vi "Turn To Angle.vi"(9 "Speed/Direction":dbl, 10 "Angle":dbl, 11 "drive.lvclass":refnum<class "drive.lvclass">) -> (3 "drive.lvclass":refnum<class "drive.lvclass">)   [LabVIEW 2015, in "drive.lvclass"]
uses:
  drive.lvclass
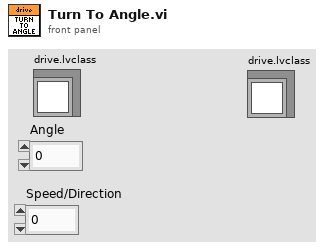
[diagram p1: front panel]
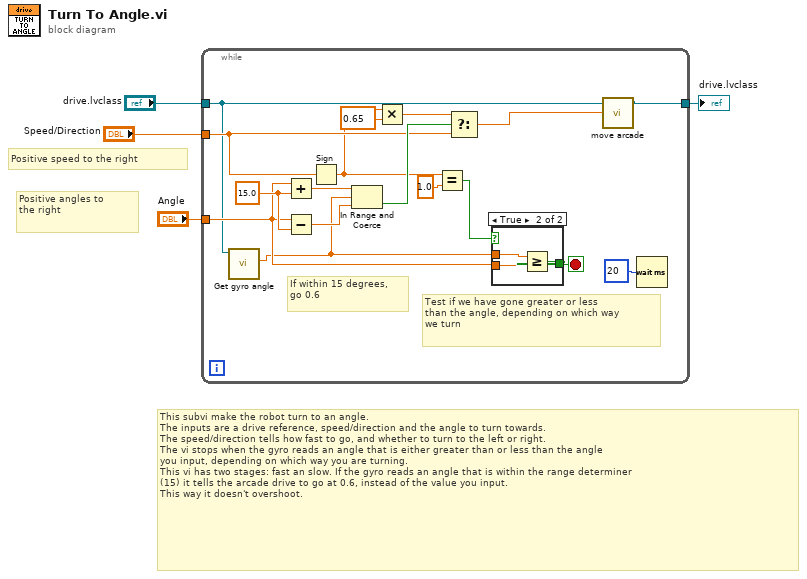
[diagram p0: block diagram]
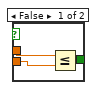
[diagram p2: hidden frame]
diagram:
  # "Positive speed to the right"
  # "Positive angles to\nthe right"
  # "This subvi make the robot turn to an angle.\nThe inputs are a drive reference, speed/direction and the angle to turn towards.\nThe speed/direction tells how fast to go, and whether to turn to the left or right.\nThe vi stops when the gyro reads an angle that is either greater than or less than the angle\nyou input, depending on which way you are turning.\nThis vi has two stages: fast an slow. If the gyro reads an angle that is within the range determiner\n(15) it tells the arcade drive to go at 0.6, instead of the value you input.\nThis way it doesn't overshoot."
  n1 = while {
    tunnel: [w7] -> w1
    tunnel: "drive.lvclass" -> [w5]
    tunnel: "Angle" -> [w11]
    tunnel: "Speed/Direction" -> [w14]
    stop <- w10 stop-if-true
    w18 = 15.0
    # "If within 15 degrees,\ngo 0.6"
    # "Test if we have gone greater or less\nthan the angle, depending on which way\nwe turn"
    n2 = call "Get gyro angle.vi"("drive in"=w5) -> ("Angle"=w6:dbl)  [unwired: 9 in, 1 out]
    n3 = Add(x=w11, y=w18) -> (x+y=w16:dbl)
    n4 = Subtract(x=w11, y=w18) -> (x-y=w17:dbl)
    n5 = Sign(1:w14) -> (0:w12:dbl)
    n6 = In Range and Coerce(upper limit=w16, x=w6, lower limit=w17) -> (In Range?=w19:bool)  [unwired: 1 out]
    n7 = Multiply(x=0.65 ("t"), y=w12) -> (x*y=w13:dbl)
    n8 = Equal?(x=w12, y=1.0) -> (x = y?=w9:bool)
    n9 = Select(t=w13, s=w19, f=w14) -> (s? t:f=w8:dbl)
    n10 = case shown="True" w9 {
      tunnel: [w24 w27] -> w10
      tunnel: w6 -> [w22 w26]
      tunnel: w11 -> [w23 w25]
      frame False {
        n11 = Less Or Equal?(x=w22, y=w23) -> (x <= y?=w24:bool)
      }
      frame True {
        n12 = Greater Or Equal?(x=w26, y=w25) -> (x >= y?=w27:bool)
      }
    }
    n13 = call "move arcade.vi"("Turn Value"=w8, "drive.lvclass"=w5) -> ("drive.lvclass"=w7:refnum<class "drive.lvclass">)  [unwired: 9 in]
    n14 = Wait (ms)(milliseconds to wait=u32 20) -> ()  [unwired: 1 out]
  }
  "drive.lvclass" <- w1
